vi "ProgressBar setRefnum.vi"(8 "error in (no error)":errorcluster, 10 "refnum":T1, 11 "ProgressBar in":refnum<class "ProgressBar.lvclass">) -> (0 "error out":errorcluster, 3 "ProgressBar out":refnum<class "ProgressBar.lvclass">)   [LabVIEW 2018, in "ProgressBar.lvclass"]
uses:
  ProgressBar.lvclass
  ProgressBar.lvclass/ProgressBar.ctl
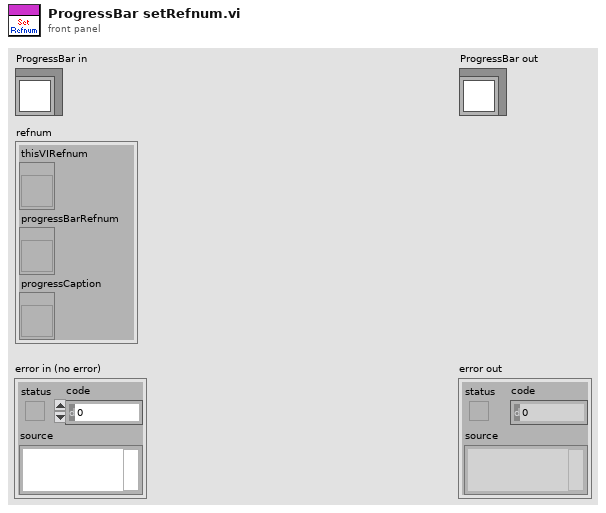
[diagram p1: front panel]
types:
  T1 = cluster{"thisVIRefnum":refnum<vi>, "progressBarRefnum":refnum<vi>, "progressCaption":refnum<vi>}
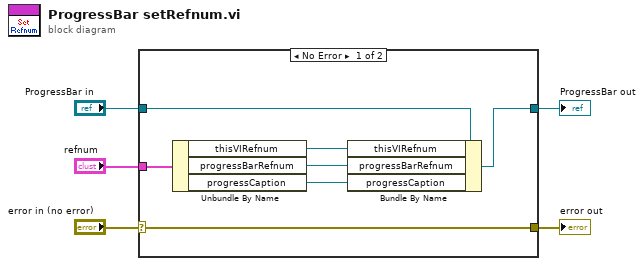
[diagram p0: block diagram]
diagram:
  n1 = case shown="No Error" "error in (no error)" {
    selector: "error in (no error)" -> [w12 w14]
    tunnel: [w12 w14] -> w4
    tunnel: [w7 w13] -> w2
    tunnel: "ProgressBar in" -> [w11 w13]
    tunnel: "refnum" -> [w10 _]
    frame No Error {
      n2 = Unbundle By Name(w10) -> ("thisVIRefnum"=w9:refnum<vi>, "progressBarRefnum"=w8:refnum<vi>, "progressCaption"=w6:refnum<vi>)
      n3 = Bundle By Name(cluster=w11, "thisVIRefnum"=w9, "progressBarRefnum"=w8, "progressCaption"=w6) -> (w7:refnum<class "ProgressBar.lvclass">)
    }
    frame Error {
    }
  }
  "error out" <- w4
  "ProgressBar out" <- w2
